vi "conversation one signal line.vi"(0 "Serial Port":refnum<visa-resource-name>, 5 "data points":u8=5, 11 "first":bool, 12 "Max time (ms)":u32=2000) -> (3 "Serial Port":refnum<visa-resource-name>, 4 "correct command":bool, 6 "command":string="SD", 8 "return code":string="PR", 10 "channel":u8=1, 13 "Time out":bool, 14 "emptied buffer":bool, 15 "return string":string)   [LabVIEW 2012]
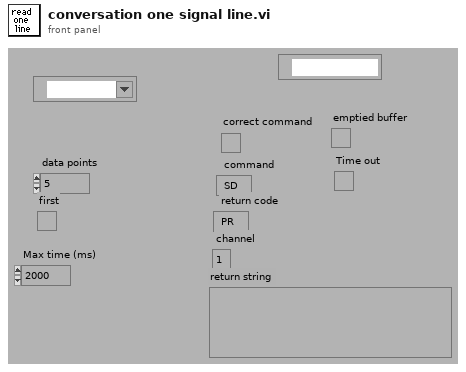
[diagram p1: front panel]
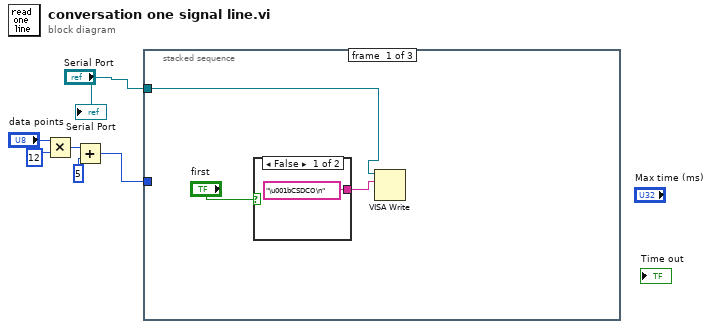
[diagram p0: block diagram]
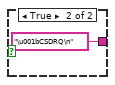
[diagram p2: hidden frame]
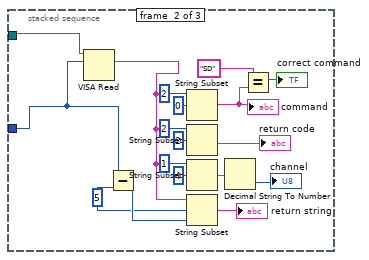
[diagram p3: hidden frame]
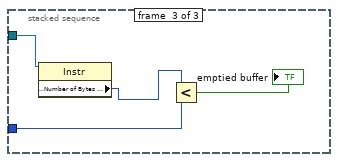
[diagram p4: hidden frame]
diagram:
  n1 = Multiply(x="data points", y=12) -> (x*y=w4:i32)
  n2 = Add(x=w4, y=5) -> (x+y=w2:i32)
  n3 = stacked-sequence {
    tunnel: "Serial Port" -> [w7 w14 w31]
    tunnel: w2 -> [_ w12 w33]
    frame #0 {
      n4 = case shown="False" "first" {
        tunnel: ["\u001bCSDCO\n" "\u001bCSDRQ\n"] -> w8
        frame False {
        }
        frame True {
        }
      }
      n5 = VISA Write(VISA resource name=w7, write buffer=w8) -> ()  [unwired: 1 in, 3 out]
    }
    frame #1 {
      w28 = 5
      n6 = VISA Read(VISA resource name=w14, byte count=w12) -> (read buffer=w13:string)  [unwired: 1 in, 3 out]
      n7 = Subtract(x=w12, y=w28) -> (x-y=w29:i32)
      n8 = String Subset(string=w13, offset (0)=0, length (rest)=2) -> (substring=w15:string)
      "command" <- w15
      n9 = String Subset(string=w13, offset (0)=2, length (rest)=2) -> (substring=→"return code":string)
      n10 = String Subset(string=w13, offset (0)=4, length (rest)=1) -> (substring=w26:string)
      n11 = String Subset(string=w13, offset (0)=w28, length (rest)=w29) -> (substring=→"return string":string)
      n12 = Decimal String To Number(string=w26) -> (number=→"channel":i32)  [unwired: 2 in, 1 out]
      n13 = Equal?(x="SD", y=w15) -> (x = y?=→"correct command":bool)
    }
    frame #2 {
      n14 = property class="Instr"(reference=w31) -> ("Serial Settings:Number of Bytes at Serial Port"=w30:u32)  [unwired: 1 in, 2 out]
      n15 = Less?(x=w30, y=w33) -> (x < y?=→"emptied buffer":bool)
    }
  }
  "Serial Port" <- "Serial Port"
